vi "Bind To Name.vi"(8 "error in (no error)":errorcluster, 10 "Type":refnum<class>, 11 "Flatten To JSON Object in":refnum<class "Flatten To JSON Object.lvclass">) -> (0 "error out":errorcluster, 2 "Type Name":string, 3 "Flatten To JSON Object out":refnum<class "Flatten To JSON Object.lvclass">)   [LabVIEW 2017, in "Flatten To JSON Object.lvclass"]
doc: "Controls the binding of a type to a serialized object."
uses:
  Flatten To JSON Object.lvclass
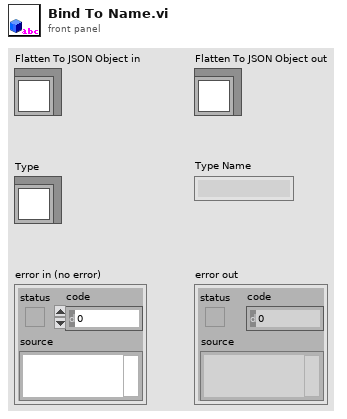
[diagram p1: front panel]
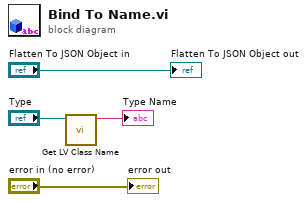
[diagram p0: block diagram]
diagram:
  n1 = call <vilib>:"Get LV Class Name.vi"("object"="Type") -> ("class name"=→"Type Name":string)  [unwired: 9 in, 1 out]
  "error out" <- "error in (no error)"
  "Flatten To JSON Object out" <- "Flatten To JSON Object in"
